vi "Zombie Left Cell String.vi"(8 "Error In":errorcluster, 10 "Bookmark ID":u32, 11 "VI Path":path) -> (0 "Error Out":errorcluster, 1 "Bold?":bool, 2 "Color":u32(colorbox)=40705, 3 "Text":string)   [LabVIEW 2017, in "Bookmark Manager.lvlib"]
doc: "Gets the left cell string for a zombie child item in the bookmarks tree. If the Spirit frame is enabled, then the text is \"Corpse\". If the Corpse frame is enabled, then the text is \"Reanimated\"."
uses:
  Bookmark Manager.lvlib
  Eulogy/Public/Typedefs/Zombie States.ctl
  Eulogy/Eulogy.lvlib
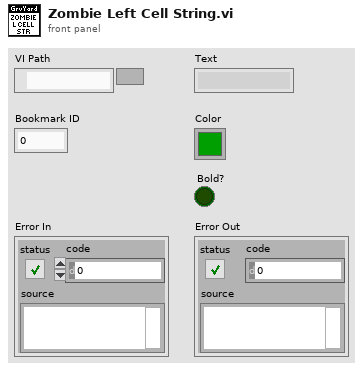
[diagram p1: front panel]
types:
  T1 = typedef "Eulogy.lvlib/Zombie States.ctl" = enum16{"Corpse", "Reanimated"}
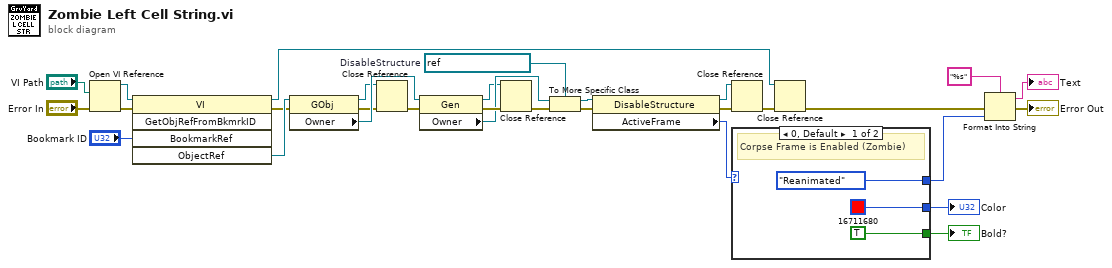
[diagram p0: block diagram]
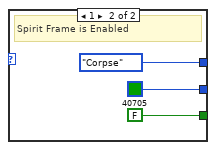
[diagram p2: hidden frame]
diagram:
  w24 = refnum<vi> refnum  # DisableStructure
  n1 = Open VI Reference(vi path="VI Path", error in (no error)="Error In") -> (vi reference=w25:refnum<vi>, error out=w26:errorcluster)  [unwired: 4 in]
  n2 = invoke class="VI" method="GetObjRefFromBkmrkID"(reference=w25, error in=w26, "BookmarkRef"="Bookmark ID") -> (reference out=w16:refnum<vi>, error out=w7:errorcluster, "ObjectRef"=w30:refnum<vi>)  [unwired: 2 in, 2 out]
  n3 = property class="GObj"(reference=w30, error in=w7) -> (reference out=w13:refnum<vi>, error out=w14:errorcluster, "Owner"=w18:refnum<vi>)
  n4 = Close Reference(reference=w13, error in (no error)=w14) -> (error out=w12:errorcluster)
  n5 = property class="Gen"(reference=w18, error in=w12) -> (reference out=w8:refnum<vi>, error out=w11:errorcluster, "Owner"=w10:refnum<vi>)
  n6 = Close Reference(reference=w8, error in (no error)=w11) -> (error out=w9:errorcluster)
  n7 = To More Specific Class(target class=w24, reference=w10, error in=w9) -> (specific class reference=w23:refnum<vi>, error out=w22:errorcluster)
  n8 = property class="DisableStructure"(reference=w23, error in=w22) -> (reference out=w19:refnum<vi>, error out=w20:errorcluster, "ActiveFrame"=w21:i16)
  n9 = Close Reference(reference=w19, error in (no error)=w20) -> (error out=w15:errorcluster)
  n10 = case shown="0, Default" w21 {
    tunnel: [Zombie_States."Reanimated" ("Zombie State") Zombie_States."Corpse" ("Zombie State")] -> w5
    tunnel: [TRUE FALSE] -> w2
    tunnel: [u32 16711680 u32 40705] -> w1
    frame 0, Default {
      # "Corpse Frame is Enabled (Zombie)"
    }
    frame 1 {
      # "Spirit Frame is Enabled"
    }
  }
  "Bold?" <- w2
  "Color" <- w1
  n11 = Close Reference(reference=w16, error in (no error)=w15) -> (error out=w17:errorcluster)
  n12 = Format Into String(format string="%s", error in=w17, w5) -> (resulting string=→"Text":string, error out=→"Error Out":errorcluster)  [unwired: 1 in]
